vi "IPS Parse Status.vi"(8 "error in (no error)":errorcluster, 10 "X String":string="X42A1C2H5M12P21\r") -> (0 "error out":errorcluster, 1 "X Strings":T1, 2 "X Cluster":T8={"System 1"=enum."Normal", "System 2"=enum."Outside Positive Current Limi", "Activity"=enum."Hold", "Switch Heater"=enum."No Switch Fitted", "Mode 1"=enum."Amps Fast", "Mode 2"=enum."At Rest"})   [LabVIEW 2016, in "IPS-120.lvlib"]
uses:
  IPS-120.lvlib
  Typedefs/Read X - Cluster.ctl
  Typedefs/Read System 1 - Enum.ctl
  Typedefs/Read System 2 - Enum.ctl
  Typedefs/Read Activity - Enum.ctl
  Typedefs/Read Switch Heater - Enum.ctl
  Typedefs/Read Mode 1 - Enum.ctl
  Typedefs/Read Mode 2 - Enum.ctl
panel:
  out "Mode 2":T2
  out "Mode 1":T3
  out "Switch Heater":T4
  out "Activity":T5
  out "System 2":T6
  out "System 1":T7
  out "System":string="42"
  out "Mode":string="12"
  out "Activity":i32=1
  out "Switch Heater":i32=5
  out "System":string="X42"
  out "Activity":string="A1"
  out "LOC/REM":string="C2"
  out "Switch Heater":string="H5"
  out "Mode":string="M12"
  out "Polarity":string="P21\r"
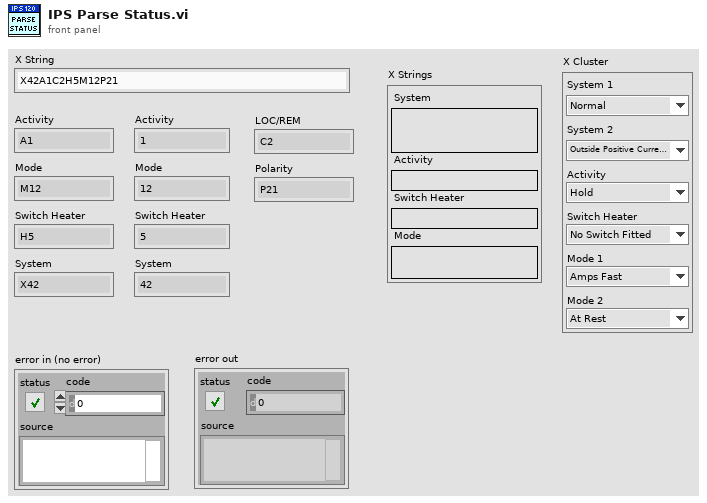
[diagram p1: front panel]
types:
  T1 = cluster{"System":string, "Activity":string, "Switch Heater":string, "Mode":string}
  T2 = typedef "IPS-120.lvlib/Read Mode 2 - Enum.ctl" = enum16{"At Rest", "Sweeping", "Sweep Limiting", "Sweeping & Sweep Limiting"}
  T3 = typedef "IPS-120.lvlib/Read Mode 1 - Enum.ctl" = enum16{"Amps Fast", "Tesla Fast", "Amps Slow", "Tesla Slow"}
  T4 = typedef "IPS-120.lvlib/Read Switch Heater - Enum.ctl" = enum16{"Off Magnet at Zero", "On", "Off Magnet at Field", "Heater Fault", "No Switch Fitted"}
  T5 = typedef "IPS-120.lvlib/Read Activity - Enum.ctl" = enum16{"Hold", "To Set Point", "To Zero", "Clamped"}
  T6 = typedef "IPS-120.lvlib/Read System 2 - Enum.ctl" = enum16{"Normal", "On Positive Voltage Limit", "On Negative Voltage Limit", "Outside Negative Current Limit", "Outside Positive Current Limi"}
  T7 = typedef "IPS-120.lvlib/Read System 1 - Enum.ctl" = enum16{"Normal", "Quenched", "Over Heated", "Warming Up", "Fault"}
  T8 = typedef "IPS-120.lvlib/Read X - Cluster.ctl" = cluster{"System 1":T7, "System 2":T6, "Activity":T5, "Switch Heater":T4, "Mode 1":T3, "Mode 2":T2}
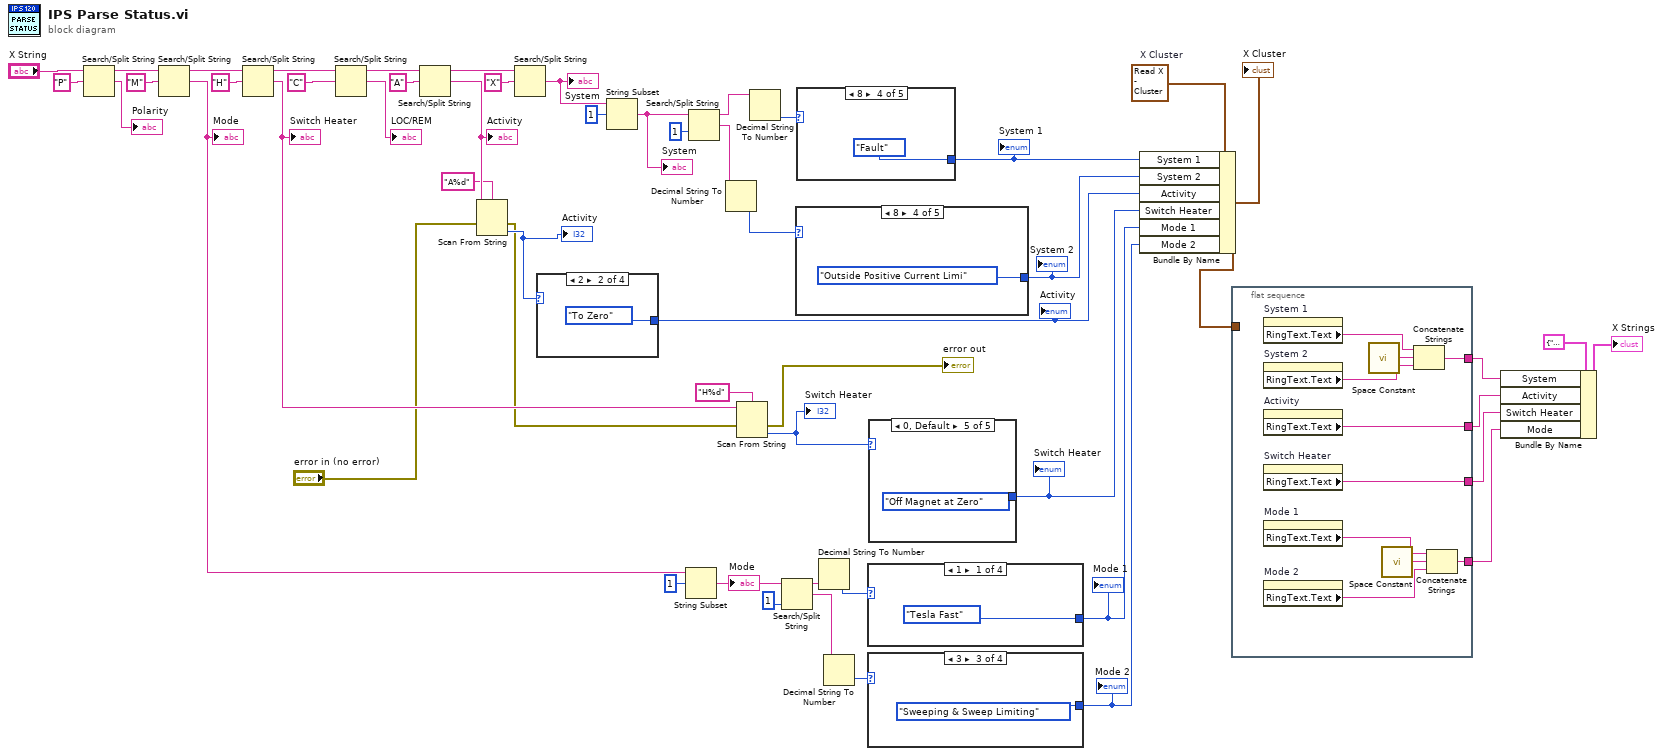
[diagram p0: block diagram]
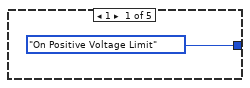
[diagram p2: hidden frame]
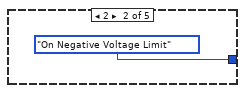
[diagram p3: hidden frame]
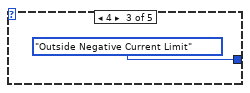
[diagram p4: hidden frame]
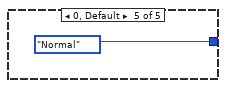
[diagram p5: hidden frame]
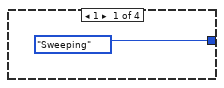
[diagram p6: hidden frame]
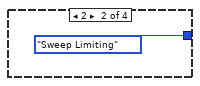
[diagram p7: hidden frame]
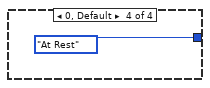
[diagram p8: hidden frame]
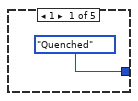
[diagram p9: hidden frame]
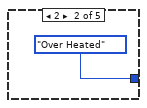
[diagram p10: hidden frame]
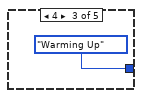
[diagram p11: hidden frame]
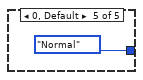
[diagram p12: hidden frame]
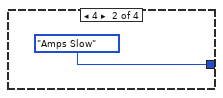
[diagram p13: hidden frame]
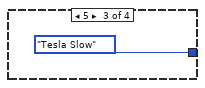
[diagram p14: hidden frame]
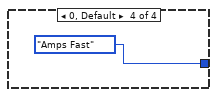
[diagram p15: hidden frame]
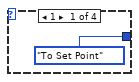
[diagram p16: hidden frame]
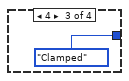
[diagram p17: hidden frame]
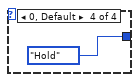
[diagram p18: hidden frame]
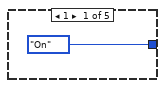
[diagram p19: hidden frame]
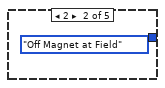
[diagram p20: hidden frame]
diagram:
  w17 = T8 {"System 1"=enum."Normal", "System 2"=enum."Outside Positive Current Limi", "Activity"=enum."Hold", "Switch Heater"=enum."No Switch Fitted", "Mode 1"=enum."Amps Fast", "Mode 2"=enum."At Rest"}  # X Cluster
  n1 = Search/Split String(string="X String", search string/char (-)="P") -> (substring before match=w50:string, match + rest of string=→"Polarity":string)  [unwired: 1 in, 1 out]
  n2 = Search/Split String(string=w50, search string/char (-)="M") -> (substring before match=w49:string, match + rest of string=w35:string)  [unwired: 1 in, 1 out]
  "Mode" <- w35
  n3 = Search/Split String(string=w49, search string/char (-)="H") -> (substring before match=w47:string, match + rest of string=w39:string)  [unwired: 1 in, 1 out]
  "Switch Heater" <- w39
  n4 = Search/Split String(string=w47, search string/char (-)="C") -> (substring before match=w45:string, match + rest of string=→"LOC/REM":string)  [unwired: 1 in, 1 out]
  n5 = Search/Split String(string=w45, search string/char (-)="A") -> (substring before match=w42:string, match + rest of string=w37:string)  [unwired: 1 in, 1 out]
  "Activity" <- w37
  n6 = Scan From String(format string="A%d", input string=w37, error in="error in (no error)") -> (error out=w2:errorcluster, output 1=w18:i32)  [unwired: 2 in, 2 out]
  "Activity" <- w18
  n7 = Search/Split String(string=w42, search string/char (-)="X") -> (match + rest of string=w32:string)  [unwired: 1 in, 2 out]
  "System" <- w32
  n8 = case shown="2" w18 {
    tunnel: [Read_Activity_-_Enum."To Set Point" ("Activity") Read_Activity_-_Enum."To Zero" ("Activity") Read_Activity_-_Enum."Clamped" ("Activity") Read_Activity_-_Enum."Hold" ("Activity")] -> w14
    frame 1 {
    }
    frame 2 {
    }
    frame 4 {
    }
    frame 0, Default {
    }
  }
  "Activity" <- w14
  n9 = String Subset(string=w32, offset (0)=1) -> (substring=w28:string)  [unwired: 1 in]
  "System" <- w28
  n10 = String Subset(string=w35, offset (0)=1) -> (substring=w19:string)  [unwired: 1 in]
  "Mode" <- w19
  n11 = Search/Split String(string=w28, offset (0)=1) -> (substring before match=w23:string, match + rest of string=w25:string)  [unwired: 1 in, 1 out]
  n12 = Decimal String To Number(string=w25) -> (number=w24:i32)  [unwired: 2 in, 1 out]
  n13 = Scan From String(format string="H%d", input string=w39, error in=w2) -> (error out=→"error out":errorcluster, output 1=w27:i32)  [unwired: 2 in, 2 out]
  "Switch Heater" <- w27
  n14 = Decimal String To Number(string=w23) -> (number=w26:i32)  [unwired: 2 in, 1 out]
  n15 = Search/Split String(string=w19, offset (0)=1) -> (substring before match=w31:string, match + rest of string=w30:string)  [unwired: 1 in, 1 out]
  n16 = case shown="8" w24 {
    tunnel: [Read_System_2_-_Enum."On Positive Voltage Limit" ("System 2") Read_System_2_-_Enum."On Negative Voltage Limit" ("System 2") Read_System_2_-_Enum."Outside Negative Current Limit" ("System 2") Read_System_2_-_Enum."Outside Positive Current Limi" ("System 2") Read_System_2_-_Enum."Normal" ("System 2")] -> w15
    frame 1 {
    }
    frame 2 {
    }
    frame 4 {
    }
    frame 8 {
    }
    frame 0, Default {
    }
  }
  "System 2" <- w15
  n17 = case shown="8" w26 {
    tunnel: [Read_System_1_-_Enum."Quenched" ("System 1") Read_System_1_-_Enum."Over Heated" ("System 1") Read_System_1_-_Enum."Warming Up" ("System 1") Read_System_1_-_Enum."Fault" ("System 1") Read_System_1_-_Enum."Normal" ("System 1")] -> w16
    frame 1 {
    }
    frame 2 {
    }
    frame 4 {
    }
    frame 8 {
    }
    frame 0, Default {
    }
  }
  "System 1" <- w16
  n18 = Decimal String To Number(string=w31) -> (number=w22:i32)  [unwired: 2 in, 1 out]
  n19 = Decimal String To Number(string=w30) -> (number=w21:i32)  [unwired: 2 in, 1 out]
  n20 = case shown="1" w22 {
    tunnel: [Read_Mode_1_-_Enum."Tesla Fast" ("Mode 1") Read_Mode_1_-_Enum."Amps Slow" ("Mode 1") Read_Mode_1_-_Enum."Tesla Slow" ("Mode 1") Read_Mode_1_-_Enum."Amps Fast" ("Mode 1")] -> w12
    frame 1 {
    }
    frame 4 {
    }
    frame 5 {
    }
    frame 0, Default {
    }
  }
  "Mode 1" <- w12
  n21 = case shown="3" w21 {
    tunnel: [Read_Mode_2_-_Enum."Sweeping" ("Mode 2") Read_Mode_2_-_Enum."Sweep Limiting" ("Mode 2") Read_Mode_2_-_Enum."Sweeping & Sweep Limiting" ("Mode 2") Read_Mode_2_-_Enum."At Rest" ("Mode 2")] -> w11
    frame 1 {
    }
    frame 2 {
    }
    frame 3 {
    }
    frame 0, Default {
    }
  }
  "Mode 2" <- w11
  n22 = case shown="0, Default" w27 {
    tunnel: [Read_Switch_Heater_-_Enum."On" ("Read Switch Heater") Read_Switch_Heater_-_Enum."Off Magnet at Field" ("Read Switch Heater") Read_Switch_Heater_-_Enum."Heater Fault" ("Read Switch Heater") Read_Switch_Heater_-_Enum."No Switch Fitted" ("Read Switch Heater") Read_Switch_Heater_-_Enum."Off Magnet at Zero" ("Read Switch Heater")] -> w13
    frame 1 {
    }
    frame 2 {
    }
    frame 5 {
    }
    frame 8 {
    }
    frame 0, Default {
    }
  }
  "Switch Heater" <- w13
  n23 = Bundle By Name(cluster=w17, "System 1"=w16, "System 2"=w15, "Activity"=w14, "Switch Heater"=w13, "Mode 1"=w12, "Mode 2"=w11) -> (w10:T8)
  "X Cluster" <- w10
  n24 = flat-sequence {
    tunnel: w10 -> [_]
    tunnel: [w84] -> w8
    tunnel: [w83] -> w5
    tunnel: [w82] -> w6
    tunnel: [w81] -> w7
    frame #0 {
      n25 = property on="System 1" class="Enum (strict)"() -> ("RingText.Text"=w89:string)  [unwired: 2 in, 2 out]
      n26 = property on="System 2" class="Enum (strict)"() -> ("RingText.Text"=w88:string)  [unwired: 2 in, 2 out]
      n27 = property on="Activity" class="Enum (strict)"() -> ("RingText.Text"=w83:string)  [unwired: 2 in, 2 out]
      n28 = property on="Switch Heater" class="Enum (strict)"() -> ("RingText.Text"=w82:string)  [unwired: 2 in, 2 out]
      n29 = property on="Mode 1" class="Enum (strict)"() -> ("RingText.Text"=w86:string)  [unwired: 2 in, 2 out]
      n30 = property on="Mode 2" class="Enum (strict)"() -> ("RingText.Text"=w85:string)  [unwired: 2 in, 2 out]
      n31 = call <vilib>:"Space Constant.vi"() -> ("String"=w90:string)
      n32 = call <vilib>:"Space Constant.vi"() -> ("String"=w87:string)
      n33 = Concatenate Strings(w89, w90, w88) -> (w84:string)
      n34 = Concatenate Strings(w86, w87, w85) -> (w81:string)
    }
  }
  n35 = Bundle By Name(cluster=T1 {"System"="", "Activity"="", "Switch Heater"="", "Mode"=""} ("X Strings 2"), "System"=w8, "Activity"=w5, "Switch Heater"=w6, "Mode"=w7) -> (→"X Strings":T1)
